vi "Set DataArray (Variant).vi"(8 "error in":errorcluster, 10 "Data":variant[][](array[variant]), 11 "DataGridView in":refnum<class "DataGridView.lvclass">) -> (0 "error out":errorcluster, 3 "DataGridView out":refnum<class "DataGridView.lvclass">)   [LabVIEW 2016, in "DataGrid.lvlib" / "DataGridView.lvclass"]
uses:
  <userlib>/LabVIEWdotNetDataGrid/source/DataGridView/DataGridView.lvclass
  <userlib>/LabVIEWdotNetDataGrid/source/DataGridView/DataGridView.lvclass/DataGridView.ctl
  System.Windows.Forms
  <userlib>/LabVIEWdotNetDataGrid/source/DataTable/Add Rows (Variant).vi
  <userlib>/LabVIEWdotNetDataGrid/source/DataTable/DataTable.lvclass
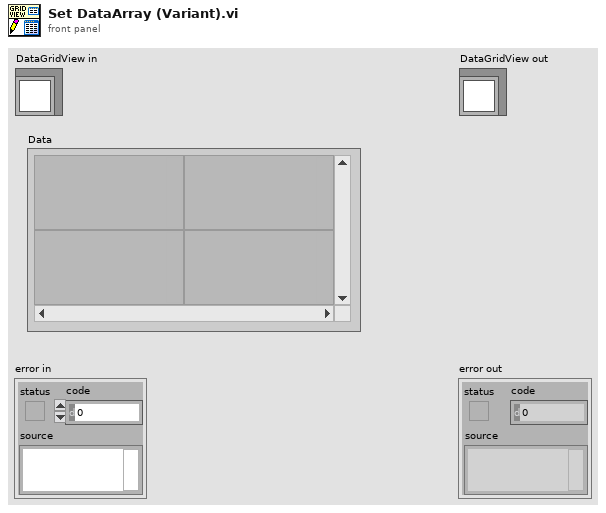
[diagram p1: front panel]
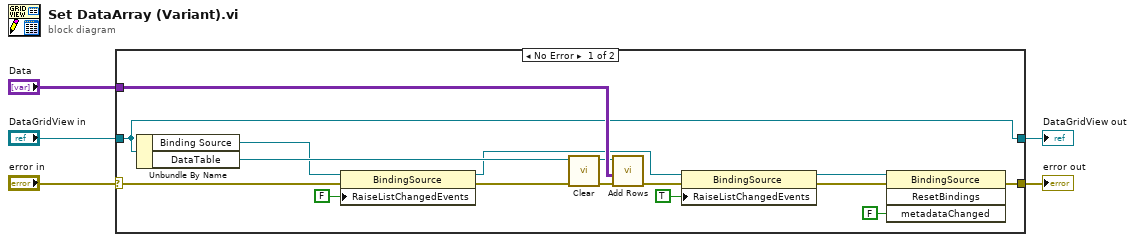
[diagram p0: block diagram]
diagram:
  n1 = case shown="No Error" "error in" {
    selector: "error in" -> [w14 w22]
    tunnel: [w11 w22] -> w4
    tunnel: [w20 w23] -> w2
    tunnel: "DataGridView in" -> [w20 w23]
    tunnel: "Data" -> [w21 _]
    frame No Error {
      n2 = Unbundle By Name(w20) -> ("Binding Source"=w16:refnum<k24>, "DataTable"=w18:refnum<class "DataTable.lvclass">)
      n3 = property class="BindingSource"(reference=w16, error in=w14, "RaiseListChangedEvents"=FALSE) -> (reference out=w15:refnum<k24>, error out=w13:errorcluster)
      n4 = call <userlib>:"Clear.vi"("error in (no error)"=w13, "DataTable in"=w18) -> ("error out"=w19:errorcluster, "DataTable out"=w17:refnum<class "DataTable.lvclass">)  [unwired: 8 in]
      n5 = call-poly <userlib>:"Add Rows.vi"("error in (no error)"=w19, "Data"=w21, "DataTable in"=w17) -> ("error out"=w12:errorcluster)  [unwired: 7 in, 1 out]
      n6 = property class="BindingSource"(reference=w15, error in=w12, "RaiseListChangedEvents"=TRUE) -> (reference out=w8:refnum<k24>, error out=w9:errorcluster)
      n7 = invoke class="BindingSource" method="ResetBindings"(reference=w8, error in=w9, "metadataChanged"=FALSE) -> (error out=w11:errorcluster)  [unwired: 1 in, 3 out]
    }
    frame Error {
    }
  }
  "error out" <- w4
  "DataGridView out" <- w2
